vi "sub_heading-data_check.vi"(11 "gps received data-arr":string[](array[string])) -> (1 "heading_str":string, 2 "heading":dbl, 3 "heading_check":bool)   [LabVIEW 2019]
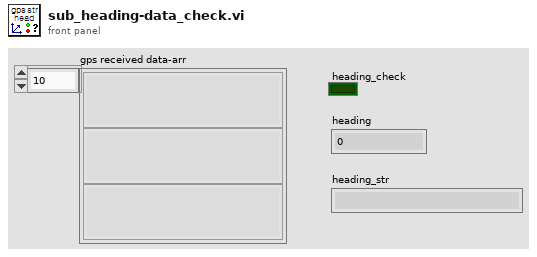
[diagram p1: front panel]
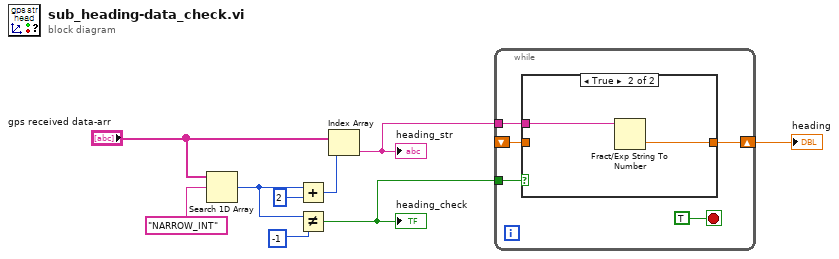
[diagram p0: block diagram]
diagram:
  n1 = Search 1D Array(1D array="gps received data-arr", element="NARROW_INT" ("盔家")) -> (index of element=w6:i32)  [unwired: 1 in]
  n2 = Add(x=w6, y=2) -> (x+y=w8:i32)
  n3 = Not Equal?(x=w6, y=-1) -> (x != y?=w3:bool)
  "heading_check" <- w3
  n4 = Index Array(array="gps received data-arr", index=w8) -> (element=w2:string)
  "heading_str" <- w2
  n5 = while {
    tunnel: w3 -> [w13]
    shift-right: [w11] -> w1
    shift-left: _ -> [w10]
    tunnel: w2 -> [w12]
    stop <- TRUE stop-if-true
    n6 = case shown="True" w13 {
      tunnel: w12 -> [_ w17]
      tunnel: [w15 w16] -> w11
      tunnel: w10 -> [w15 _]
      frame False {
      }
      frame True {
        n7 = Fract/Exp String To Number(string=w17) -> (number=w16:dbl)  [unwired: 3 in, 1 out]
      }
    }
  }
  "heading" <- w1
